vi "Oriental_step_motor_PKP225.vi"(6 "F_Threshold":fxp<+,12,12>, 8 "dFmr":fxp<+/-,25,15>, 10 "omega":fxp<+/-,20,9>, 11 "Fmr":fxp<+/-,21,11>) -> (1 "vq_F":fxp<+/-,20,5> format="%.57g", 3 "vd_F":fxp<+/-,20,5>)   [LabVIEW 2014]
uses:
  <vilib>/rvi/FXPMathLib/FxpMul/XNode/nifxpmath_Multiplier.xnode
  <vilib>/rvi/FXPMathLib/FxpAdd/XNode/nifxpmath_Add.xnode
  <vilib>/rvi/FXPMathLib/sim/FxpSim.dll
panel:
  out "Lmdtau_mr/Km":fxp<+/-,30,15>
  out "-RKm/NrL":fxp<+/-,18,3>=-1.9615478515625
  out "tauR/Km":fxp<+/-,30,15>
  out "Kmw":fxp<+/-,25,10> format="%.50g"
  out "-NrLwtau/Km":fxp<+/-,28,9> format="%.54g"
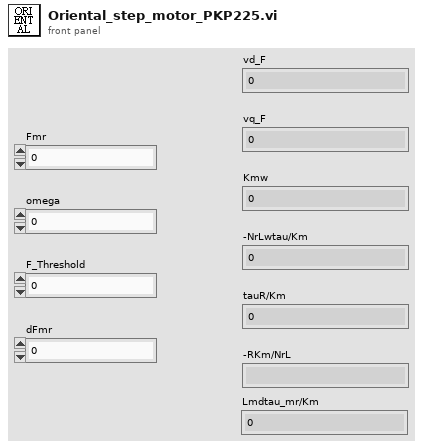
[diagram p1: front panel]
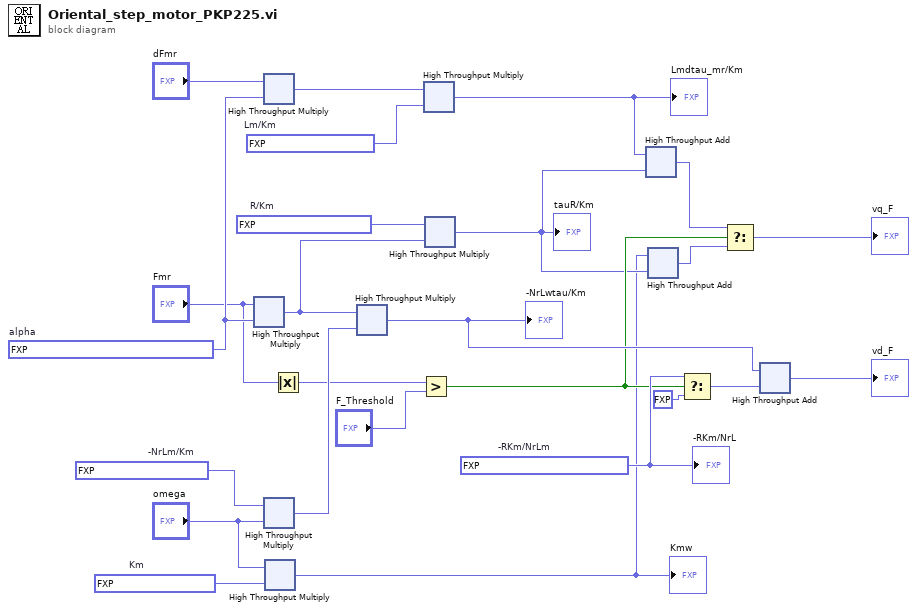
[diagram p0: block diagram]
diagram:
  w20 = fxp<+,23,7> 0.0212249755859375  # Lm/Km
  w16 = fxp<+/-,20,4> -1.0612945556640625  # -NrLm/Km
  w14 = fxp<+/-,25,4> -1.951387882232666  # -RKm/NrLm
  w22 = fxp<+,23,7> 36.26969909667969  # R/Km
  w11 = fxp<+,14,-2> 0.057098388671875  # Km
  w17 = fxp<+/-,28,0> 0.0003183111548423767  # alpha
  n1 = xnode ("High Throughput Multiply")("x"="Fmr", "y"=w17) -> ("x*y"=w12:fxp<+/-,28,9>)
  n2 = xnode ("High Throughput Multiply")("x"="dFmr", "y"=w17) -> ("x*y"=w13:fxp<+/-,28,9>)
  n3 = xnode ("High Throughput Multiply")("x"=w16, "y"="omega") -> ("x*y"=w15:fxp<+/-,28,9>)
  n4 = xnode ("High Throughput Multiply")("x"="omega", "y"=w11) -> ("x*y"=w1:fxp<+/-,22,7>)
  "Kmw" <- w1
  n5 = Absolute Value(x="Fmr") -> (abs(x)=w8:fxp<+,21,11>)
  n6 = xnode ("High Throughput Multiply")("x"=w12, "y"=w15) -> ("x*y"=w6:fxp<+/-,28,9>)
  "-NrLwtau/Km" <- w6
  n7 = Greater?(x=w8, y="F_Threshold") -> (0:w4:bool)
  n8 = xnode ("High Throughput Multiply")("x"=w13, "y"=w20) -> ("x*y"=w19:fxp<+/-,20,5>)
  "Lmdtau_mr/Km" <- w19
  n9 = xnode ("High Throughput Multiply")("x"=w22, "y"=w12) -> ("x*y"=w2:fxp<+/-,20,5>)
  "tauR/Km" <- w2
  n10 = xnode ("High Throughput Add")("x"=w19, "y"=w2) -> ("x+y"=w21:fxp<+/-,20,5>)
  n11 = xnode ("High Throughput Add")("x"=w1, "y"=w2) -> ("x+y"=w3:fxp<+/-,20,5>)
  n12 = Select(t=w14, s=w4, f=fxp<+/-,18,3> 0.0) -> (s? t:f=w5:fxp<+/-,25,4>)
  n13 = Select(t=w21, s=w4, f=w3) -> (s? t:f=→"vq_F":fxp<+/-,20,5>)
  n14 = xnode ("High Throughput Add")("x"=w6, "y"=w5) -> ("x+y"=→"vd_F":fxp<+/-,20,5>)
  "-RKm/NrL" <- w14
